vi "Get Slot Number.vi"(0 "Board Type":string) -> (1 "Number of Boards Found":i16, 2 "Slot Number(s)":u32[](array[numeric]))   [LabVIEW 2019]
doc: "Looks for the specified board type and returns Number of Boards Found and their Slot Number(s). If no boards of that type are found, then Number of Boards Found is 0 and Slot Number(s) is empty. Uses Board_ID subVI, also available in the LabDriver board-specific VIs folder."
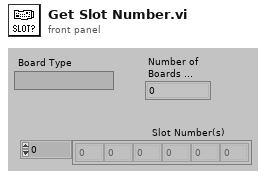
[diagram p1: front panel]
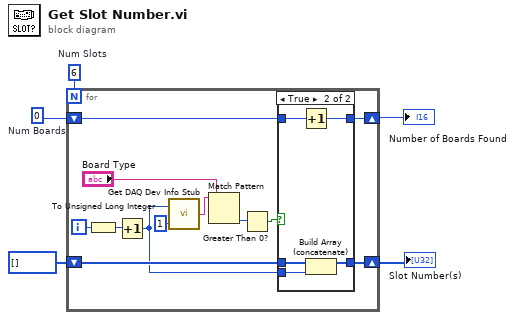
[diagram p0: block diagram]
diagram:
  w5 = 6  # Num Slots
  w2 = i16 0  # Num Boards
  n1 = for {
    N: w5 -> [_]
    shift-right: [w14] -> w3
    shift-left: u32[] [] -> [w15]
    shift-right: [w12] -> w4
    shift-left: w2 -> [w13]
    i -> [w11]
    n2 = To Unsigned Long Integer(number=w11) -> (unsigned 32bit integer=w10:u32)
    n3 = Increment(x=w10) -> (x+1=w8:u32)
    n4 = call "Get DAQ Dev Info Stub.vi"("Numeric"=u32 1, "Numeric 2"=w8) -> ("information string"=w9:string)
    n5 = Match Pattern(string=w9, regular expression="Board Type") -> (offset past match=w17:i32)  [unwired: 1 in, 3 out]
    n6 = Greater Than 0?(x=w17) -> (x > 0?=w16:bool)
    n7 = case shown="True" w16 {
      tunnel: [w18 w20] -> w12
      tunnel: w13 -> [w18 w21]
      tunnel: [w19 w22] -> w14
      tunnel: w15 -> [w19 w24]
      tunnel: w8 -> [_ w23]
      frame False {
      }
      frame True {
        n8 = Increment(x=w21) -> (x+1=w20:i16)
        n9 = Build Array (concatenate)(w24, w23) -> (w22:u32[])
      }
    }
  }
  "Number of Boards Found" <- w4
  "Slot Number(s)" <- w3
